vi "TCP_comms_receive.vi"() -> ()   [LabVIEW 2018]
panel:
  out "Sent i":i32
  out "Waveform Chart":i32(graph)
  in  "address":string="127.0.0.1"
  in  "Send many":bool
  in  "Value to send":u32
  in  "Send single value":bool
  out "Received value/i":u32
  out "Connection opened?":bool
  out "Error Out":errorcluster
  in  "Stop and Exit":bool
  in  "Error In":errorcluster
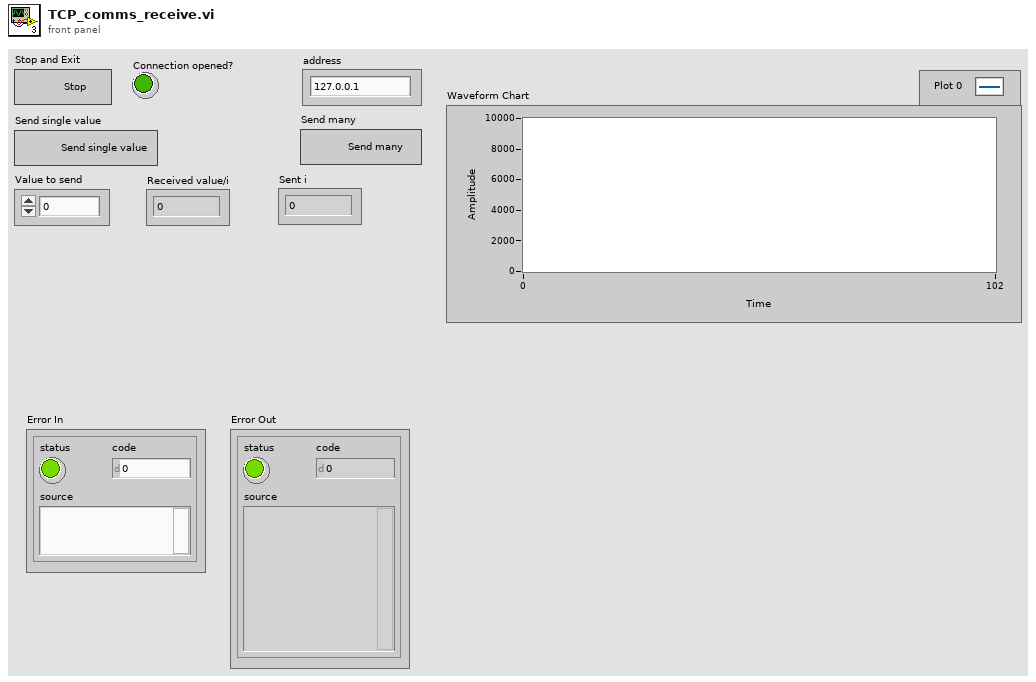
[diagram p1: front panel]
types:
  T1 = enum16{"Standard", "Buffered", "CRLF", "Immediate"}
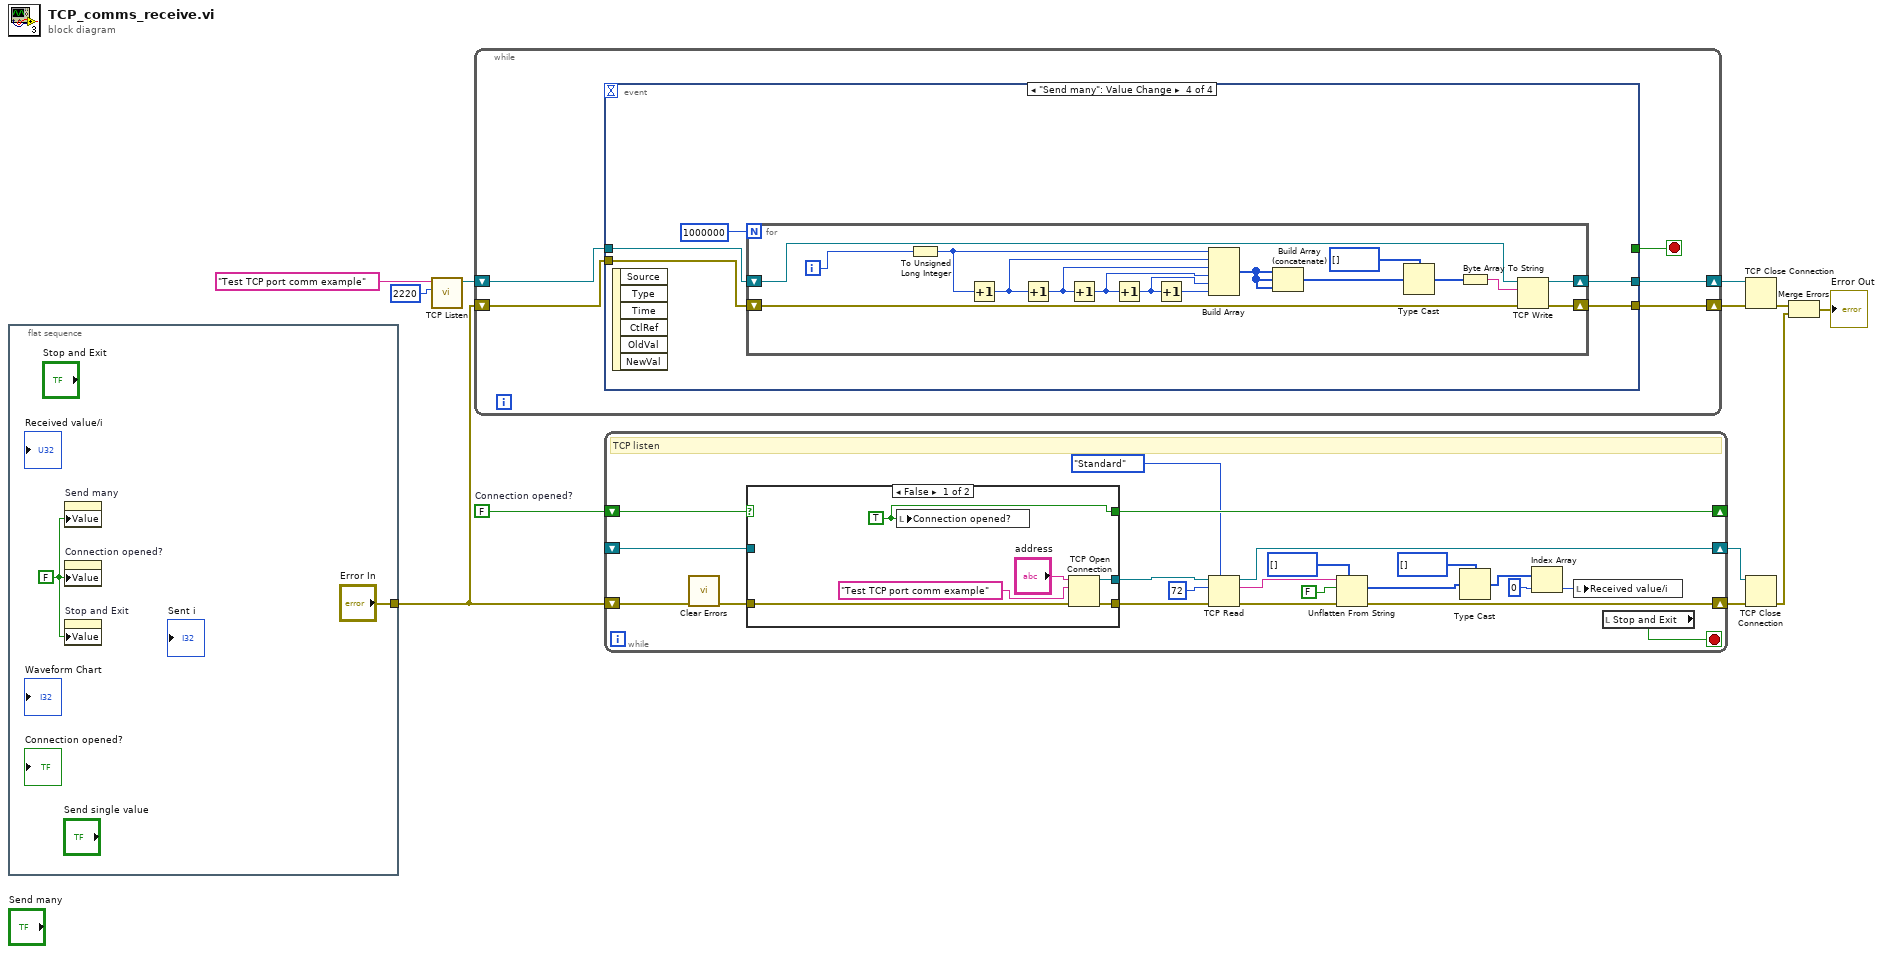
[diagram p0: block diagram]
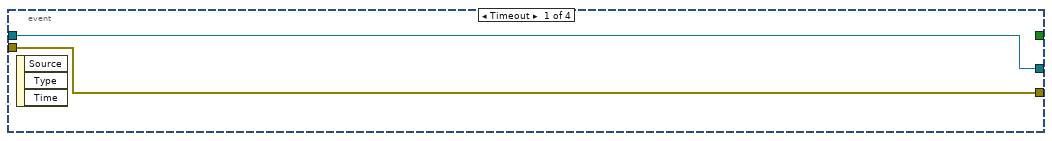
[diagram p3: hidden frame]
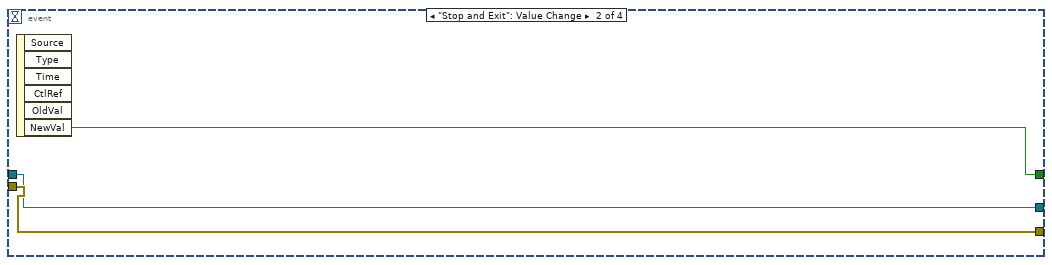
[diagram p4: hidden frame]
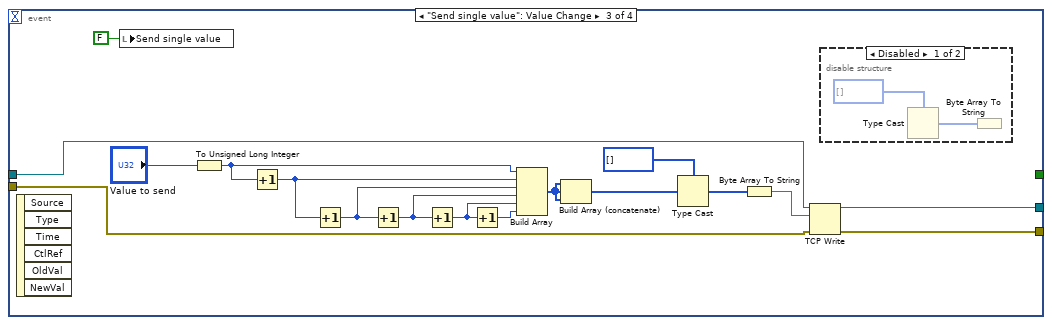
[diagram p5: hidden frame]
diagram:
  w8 = FALSE  # Connection opened?
  n1 = flat-sequence {
    tunnel: ["Error In"] -> w12
    frame #0 {
      w13 = FALSE ("Stop and Exit")
      n2 = property on="Send many" class="Bool (strict)"("Value"=w13) -> ()  [unwired: 2 in, 2 out]
      n3 = property on="Connection opened?" class="Bool (strict)"("Value"=w13) -> ()  [unwired: 2 in, 2 out]
      n4 = property on="Stop and Exit" class="Bool (strict)"("Value"=w13) -> ()  [unwired: 2 in, 2 out]
    }
  }
  n5 = call <vilib>:"TCP Listen.vi"("port"=u16 2220, "service name"="Test TCP port comm example") -> ("connection ID"=w1:refnum<k5>)  [unwired: 5 in, 4 out]
  n6 = while {
    shift-right: [w17] -> w7
    shift-left: w12 -> [w18]
    shift-right: [w15] -> w6
    shift-left: w1 -> [w16]
    stop <- w19 stop-if-true
    n7 = event shown="[3] \"Send many\": Value Change" {
      selector: _ -> [_ _ _ _]
      dyn-events: _ -> [_ _ _ _]
      timeout: _ -> [_ _ _ _]
      tunnel: [_ w24 _ _] -> w19
      tunnel: w18 -> [w21 w23 w39 w47]
      tunnel: [w21 w23 w38 w46] -> w17
      tunnel: w16 -> [w20 w22 w41 w49]
      tunnel: [w20 w22 w40 w48] -> w15
      event Timeout {
        n8 = event-data() -> ()  [unwired: 1 in, 3 out]
      }
      event "Stop and Exit": Value Change {
        n9 = event-data() -> ("NewVal"=w24:bool)  [unwired: 1 in, 5 out]
      }
      event "Send single value": Value Change {
        n10 = event-data() -> ()  [unwired: 1 in, 6 out]
        n11 = local write "Send single value"(FALSE ("Send single value")) -> ()
        n12 = To Unsigned Long Integer(number="Value to send") -> (unsigned 32bit integer=w33:u32)
        n13 = Increment(x=w33) -> (x+1=w32:u32)
        n14 = Increment(x=w32) -> (x+1=w31:u32)
        n15 = Increment(x=w31) -> (x+1=w30:u32)
        n16 = Increment(x=w30) -> (x+1=w29:u32)
        n17 = Increment(x=w29) -> (x+1=w28:u32)
        n18 = Build Array(w33, w32, w31, w30, w29, w28) -> (w26:u32[])
        n19 = Build Array (concatenate)(w26, w26, w26) -> (w25:u32[])
        n20 = Type Cast(type=u8[] [], x=w25) -> (*(type *) &x=w36:u8[])
        n21 = Byte Array To String(unsigned byte array=w36) -> (string=w35:string)
        n22 = TCP Write(connection ID=w41, data in=w35, error in (no error)=w39) -> (connection ID out=w40:refnum<k5>, error out=w38:errorcluster)  [unwired: 1 in, 1 out]
        n23 = disable-structure shown="Disabled" {
          frame Disabled {
            n24 = Type Cast(type=u8[] []) -> (x=w44:ext, *(type *) &x=w43:u8[])
            n25 = Byte Array To String(unsigned byte array=w43) -> ()  [unwired: 1 out]
          }
          frame Enabled {
          }
        }
      }
      event "Send many": Value Change {
        n26 = event-data() -> ()  [unwired: 1 in, 6 out]
        n27 = for {
          N: 1000000 -> [_]
          shift-right: [w64] -> w48
          shift-left: w49 -> [w65]
          shift-right: [w62] -> w46
          shift-left: w47 -> [w63]
          i -> [w58]
          n28 = To Unsigned Long Integer(number=w58) -> (unsigned 32bit integer=w57:u32)
          n29 = Increment(x=w57) -> (x+1=w56:u32)
          n30 = Increment(x=w56) -> (x+1=w55:u32)
          n31 = Increment(x=w55) -> (x+1=w54:u32)
          n32 = Increment(x=w54) -> (x+1=w53:u32)
          n33 = Increment(x=w53) -> (x+1=w52:u32)
          n34 = Build Array(w57, w56, w55, w54, w53, w52) -> (w51:u32[])
          n35 = Build Array (concatenate)(w51, w51, w51) -> (w50:u32[])
          n36 = Type Cast(type=u8[] [], x=w50) -> (*(type *) &x=w60:u8[])
          n37 = Byte Array To String(unsigned byte array=w60) -> (string=w59:string)
          n38 = TCP Write(connection ID=w65, data in=w59, error in (no error)=w63) -> (connection ID out=w64:refnum<k5>, error out=w62:errorcluster)  [unwired: 1 in, 1 out]
        }
      }
    }
  }
  n39 = while {
    shift-right: [w70] -> w10
    shift-left: w12 -> [w72]
    shift-right: [w84] -> _
    shift-left: w8 -> [w85]
    shift-right: [w80] -> w5
    shift-left: _ -> [w83]
    stop <- w86 stop-if-true
    # "TCP listen"
    n40 = call <vilib>:"Clear Errors.vi"("error in (no error)"=w72) -> ("error out"=w69:errorcluster)  [unwired: 5 in, 1 out]
    n41 = case shown="False" w85 {
      selector: w85 -> [_ w94]
      tunnel: w69 -> [w92 w95]
      tunnel: [w91 w95] -> w82
      tunnel: [w87 w94] -> w84
      tunnel: [w90 w93] -> w81
      tunnel: w83 -> [_ w93]
      frame False {
        w87 = TRUE
        n42 = local write "Connection opened?"(w87) -> ()
        n43 = TCP Open Connection(address="address", remote port or service name="Test TCP port comm example" ("service name"), error in (no error)=w92) -> (connection ID=w90:refnum<k5>, error out=w91:errorcluster)  [unwired: 2 in]
      }
      frame True {
      }
    }
    n44 = TCP Read(connection ID=w81, bytes to read=72, error in (no error)=w82, 7:T1."Standard" ("mode (standard)")) -> (connection ID out=w80:refnum<k5>, data out=w79:string, error out=w78:errorcluster)  [unwired: 1 in]
    n45 = Unflatten From String(type=u8[] [], binary string=w79, data includes array or string size? (T)=FALSE, error in (no error)=w78) -> (value=w75:u8[], error out=w70:errorcluster)  [unwired: 1 in, 1 out]
    n46 = Type Cast(type=u32[] [] ("*(type *) &x"), x=w75) -> (*(type *) &x=w76:u32[])
    n47 = Index Array(array=w76, index=0) -> (element=w67:u32)
    n48 = local write "Received value/i"(w67) -> ()
    n49 = local read "Stop and Exit"() -> (w86:bool)
  }
  n50 = TCP Close Connection(connection ID=w6, error in (no error)=w7) -> (error out=w4:errorcluster)  [unwired: 1 in, 1 out]
  n51 = TCP Close Connection(connection ID=w5, error in (no error)=w10) -> (error out=w9:errorcluster)  [unwired: 1 in, 1 out]
  n52 = Merge Errors(w4, w9) -> (→"Error Out":errorcluster)
